vi "VDH-handleTempCalibSet.vi"(8 "error in (no error)":errorcluster, 11 "VDH-VNA_data_handler in":refnum<class "VDH-VNA_data_handler.lvclass">) -> (0 "error out":errorcluster, 3 "VDH-VNA_data_handler out":refnum<class "VDH-VNA_data_handler.lvclass">)   [LabVIEW 2020, in "VDH-VNA_data_handler.lvlib" / "VDH-VNA_data_handler.lvclass"]
uses:
  VDH-VNA_data_handler.lvclass
  VDH-VNA_data_handler.lvclass/VDH-VNA_data_handler.ctl
  <vilib>/Analysis/baseanly.llb/Mean (CDB).vi
  <vilib>/Analysis/NI_AALBase.lvlib
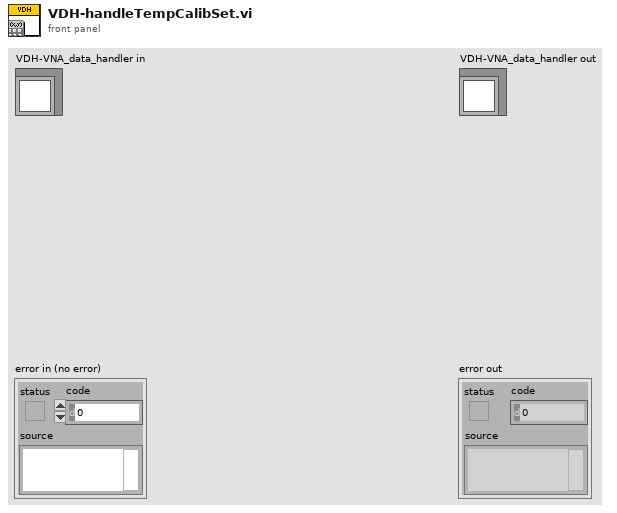
[diagram p1: front panel]
types:
  T1 = typedef "VDH-VNA_data_handler.lvlib/VDH-VNA_data_handler.lvclass/VDH-Calibration_enum.ctl" = enum16{"Non", "Short", "Open", "Load", "Through", "Permativity"}
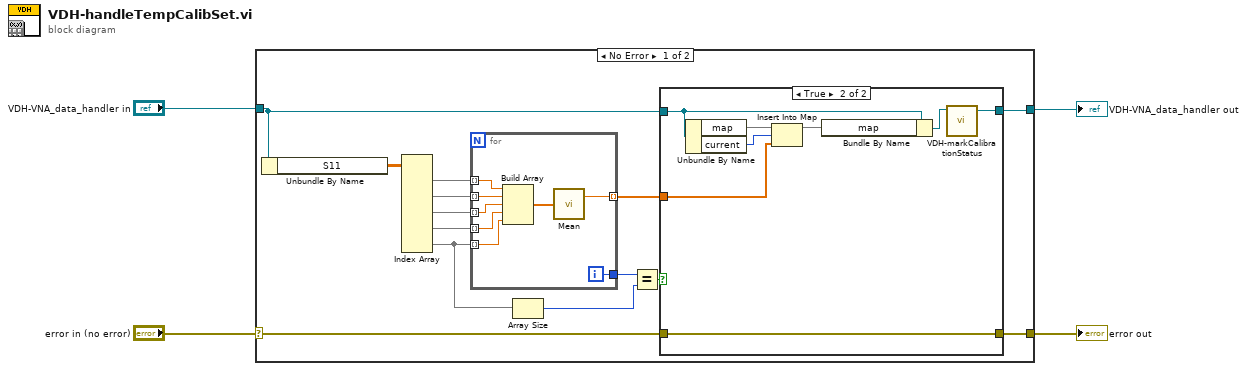
[diagram p0: block diagram]
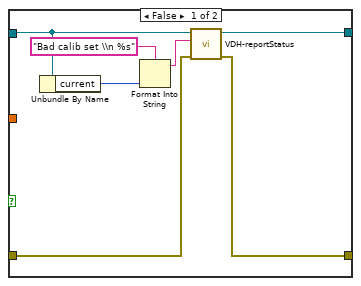
[diagram p2: hidden frame]
diagram:
  n1 = case shown="No Error" "error in (no error)" {
    selector: "error in (no error)" -> [w6 w43]
    tunnel: [w5 w43] -> w3
    tunnel: [w8 w42] -> w1
    tunnel: "VDH-VNA_data_handler in" -> [w10 w42]
    frame No Error {
      n2 = Unbundle By Name(w10) -> ("S11"=w18:cdb[][])
      n3 = Index Array(array=w18) -> (element #1=w17:cdb[], element #2=w16:cdb[], element #3=w15:cdb[], element #4=w14:cdb[], element #5=w13:cdb[])  [unwired: 10 in]
      n4 = for {
        tunnel: w17 -> [w40] mode=indexing
        tunnel: w16 -> [w39] mode=indexing
        tunnel: w15 -> [w38] mode=indexing
        tunnel: w14 -> [w37] mode=indexing
        tunnel: w13 -> [w36] mode=indexing
        tunnel: [w41] -> w11
        tunnel: [w34] -> w9 mode=indexing
        i -> [w41]
        n5 = Build Array(w40, w39, w38, w37, w36) -> (w35:cdb[])
        n6 = call-poly <vilib>:"Mean.vi"("X"=w35) -> ("mean"=w34:cdb)  [unwired: 1 out]
      }
      n7 = Array Size(array=w13) -> (size(s)=w12:i32)
      n8 = Equal?(x=w11, y=w12) -> (x = y?=w7:bool)
      n9 = case shown="True" w7 {
        tunnel: w10 -> [w22 w33]
        tunnel: w9 -> [_ w29]
        tunnel: [w25 w26] -> w8
        tunnel: w6 -> [w24 w28]
        tunnel: [w23 w28] -> w5
        frame False {
          n10 = Unbundle By Name(w22) -> ("current"=w20:T1)
          n11 = Format Into String(format string="Bad calib set \\n %s" ("message"), w20) -> (resulting string=w19:string)  [unwired: 2 in, 1 out]
          n12 = call "VDH-reportStatus.vi"("error in (no error)"=w24, "message"=w19, "VDH-VNA_data_handler in"=w22) -> ("error out"=w23:errorcluster, "VDH-VNA_data_handler out"=w25:refnum<class "VDH-VNA_data_handler.lvclass">)  [unwired: 7 in]
        }
        frame True {
          n13 = Unbundle By Name(w33) -> ("map"=w32:map{T1, cdb[]}, "current"=w30:T1)
          n14 = Insert Into Map(map in=w32, key=w30, value=w29) -> (map out=w31:map{T1, cdb[]})  [unwired: 2 out]
          n15 = Bundle By Name(cluster=w33, "map"=w31) -> (w27:refnum<class "VDH-VNA_data_handler.lvclass">)
          n16 = call "VDH-markCalibrationStatus.vi"("VDH-VNA_data_handler in"=w27) -> ("VDH-VNA_data_handler out"=w26:refnum<class "VDH-VNA_data_handler.lvclass">)  [unwired: 10 in]
        }
      }
    }
    frame Error {
    }
  }
  "error out" <- w3
  "VDH-VNA_data_handler out" <- w1
